vi "gentec-M-Link.Parse Data.vi"(1 "Data Bytes":string, 3 "Measurement":T1 items=["other Mode", "Energymode"]) -> (14 "ADC Counts":u16, 15 "Range":T2 items=["1f", "3f", "10f", "30f", "100f", "300f", "1p", "3p", "10p", "30p", "100p", "300p", "1n", "3n", "10n", "30n", "100n", "300n", "1u", "3u", "10u", "30u", "100u", "300u", "1m", "3m", "10m", "30m", "100m", "300m", "1", "3", "10", "30", "100", "300", "1K", "3K", "10K", "30K", "100K", "300K", "1M", "3M", "10M", "30M", "100M", "300M"], 16 "Pulse Period Counts":u32, 17 "new SSE":bool, 18 "Out":bool)   [LabVIEW 2014, in "gentec-M-Link - Driver.lvlib"]
uses:
  gentec-M-Link - Driver.lvlib
  Type Defs/gentec-M-Link.Range.ctl
  Type Defs/gentec-M-Link.Measurement Mode.ctl
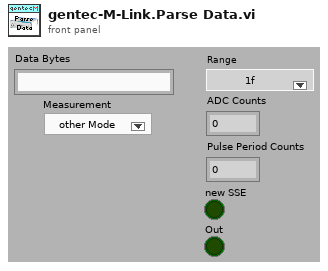
[diagram p1: front panel]
types:
  T1 = typedef "gentec-M-Link - Driver.lvlib/gentec-M-Link.Measurement Mode.ctl" = u16
  T2 = typedef "gentec-M-Link - Driver.lvlib/gentec-M-Link.Range.ctl" = u16
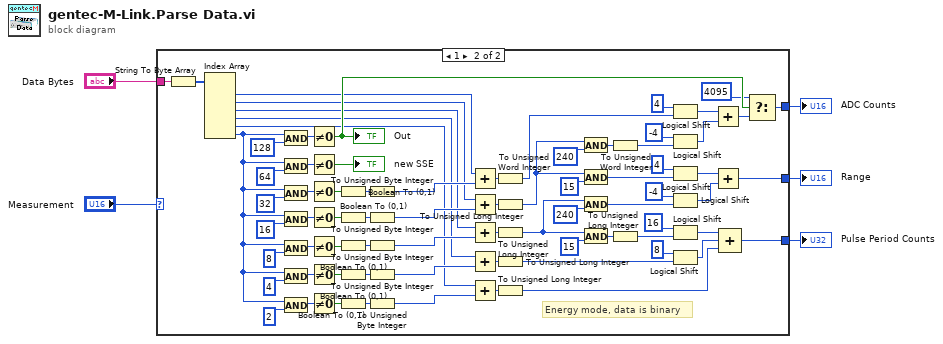
[diagram p0: block diagram]
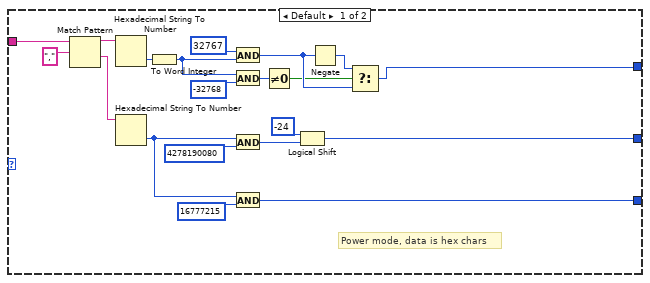
[diagram p2: hidden frame]
diagram:
  n1 = case shown="1" "Measurement" {
    tunnel: [w17 w100] -> w3
    tunnel: [w8 w99] -> w1
    tunnel: [w7 w101] -> w2
    tunnel: "Data Bytes" -> [w6 w98]
    frame Default {
      # "Power mode, data is hex chars"
      n2 = Match Pattern(string=w6, regular expression=",") -> (before substring=w24:string, after substring=w23:string)  [unwired: 3 out]
      n3 = Hexadecimal String To Number(string=w24) -> (number=w9:u32)  [unwired: 3 out]
      n4 = Hexadecimal String To Number(string=w23) -> (number=w21:u32)  [unwired: 3 out]
      n5 = To Word Integer(number=w9) -> (16bit integer=w16:i16)
      n6 = And(x=i16 32767 ("y"), y=w16) -> (x .and. y?=w15:i16)
      n7 = And(x=w16, y=i16 -32768) -> (x .and. y?=w11:i16)
      n8 = And(x=w21, y=u32 4278190080) -> (x .and. y?=w19:u32)
      n9 = And(x=w21, y=u32 16777215) -> (x .and. y?=w8:u32)
      n10 = Not Equal To 0?(x=w11) -> (x != 0?=w13:bool)
      n11 = Logical Shift(y=i8 -24, x=w19) -> (x << y=w7:u32)
      n12 = Negate(x=w15) -> (-x=w14:i16)
      n13 = Select(t=w14, s=w13, f=w15) -> (s? t:f=w17:i16)
    }
    frame 1 {
      # "Energy mode, data is binary"
      n14 = String To Byte Array(string=w98) -> (unsigned byte array=w66:u8[])
      n15 = Index Array(array=w66) -> (element #1=w33:u8, element #2=w30:u8, element #3=w29:u8, element #4=w28:u8, element #5=w26:u8, element #6=w27:u8)  [unwired: 6 in]
      n16 = And(x=w27, y=u8 128) -> (x .and. y?=w90:u8)
      n17 = And(x=w27, y=u8 64) -> (x .and. y?=w73:u8)
      n18 = And(x=w27, y=u8 32) -> (x .and. y?=w88:u8)
      n19 = And(x=w27, y=u8 16) -> (x .and. y?=w86:u8)
      n20 = And(x=w27, y=u8 8) -> (x .and. y?=w82:u8)
      n21 = And(x=w27, y=u8 4) -> (x .and. y?=w80:u8)
      n22 = And(x=w27, y=u8 2) -> (x .and. y?=w76:u8)
      n23 = Not Equal To 0?(x=w90) -> (x != 0?=w97:bool)
      "Out" <- w97
      n24 = Not Equal To 0?(x=w73) -> (x != 0?=→"new SSE":bool)
      n25 = Not Equal To 0?(x=w88) -> (x != 0?=w85:bool)
      n26 = Not Equal To 0?(x=w86) -> (x != 0?=w84:bool)
      n27 = Not Equal To 0?(x=w82) -> (x != 0?=w79:bool)
      n28 = Not Equal To 0?(x=w80) -> (x != 0?=w78:bool)
      n29 = Not Equal To 0?(x=w76) -> (x != 0?=w75:bool)
      n30 = Boolean To (0,1)(Boolean=w85) -> (0, 1=w71:i16)
      n31 = Boolean To (0,1)(Boolean=w84) -> (0, 1=w70:i16)
      n32 = Boolean To (0,1)(Boolean=w79) -> (0, 1=w69:i16)
      n33 = Boolean To (0,1)(Boolean=w78) -> (0, 1=w68:i16)
      n34 = Boolean To (0,1)(Boolean=w75) -> (0, 1=w67:i16)
      n35 = To Unsigned Byte Integer(number=w71) -> (unsigned 8bit integer=w96:u8)
      n36 = To Unsigned Byte Integer(number=w70) -> (unsigned 8bit integer=w95:u8)
      n37 = To Unsigned Byte Integer(number=w69) -> (unsigned 8bit integer=w94:u8)
      n38 = To Unsigned Byte Integer(number=w68) -> (unsigned 8bit integer=w93:u8)
      n39 = To Unsigned Byte Integer(number=w67) -> (unsigned 8bit integer=w92:u8)
      n40 = Add(x=w33, y=w96) -> (x+y=w40:u8)
      n41 = Add(x=w30, y=w95) -> (x+y=w37:u8)
      n42 = Add(x=w29, y=w94) -> (x+y=w35:u8)
      n43 = Add(x=w28, y=w93) -> (x+y=w39:u8)
      n44 = Add(x=w26, y=w92) -> (x+y=w38:u8)
      n45 = To Unsigned Word Integer(number=w40) -> (unsigned 16bit integer=w51:u16)
      n46 = To Unsigned Long Integer(number=w37) -> (unsigned 32bit integer=w36:u32)
      n47 = To Unsigned Long Integer(number=w35) -> (unsigned 32bit integer=w34:u32)
      n48 = To Unsigned Long Integer(number=w39) -> (unsigned 32bit integer=w44:u32)
      n49 = To Unsigned Long Integer(number=w38) -> (unsigned 32bit integer=w41:u32)
      n50 = And(x=w36, y=u8 240) -> (x .and. y?=w50:u32)
      n51 = And(x=w36, y=u8 15) -> (x .and. y?=w57:u32)
      n52 = And(x=w34, y=u8 240) -> (x .and. y?=w56:u32)
      n53 = And(x=w34, y=u8 15) -> (x .and. y?=w48:u32)
      n54 = To Unsigned Word Integer(number=w50) -> (unsigned 16bit integer=w49:u16)
      n55 = To Unsigned Long Integer(number=w48) -> (unsigned 32bit integer=w46:u32)
      n56 = Logical Shift(y=i8 4, x=w51) -> (x << y=w52:u16)
      n57 = Logical Shift(y=i8 -4, x=w49) -> (x << y=w53:u16)
      n58 = Logical Shift(y=i8 4, x=w57) -> (x << y=w63:u32)
      n59 = Logical Shift(y=i8 -4, x=w56) -> (x << y=w62:u32)
      n60 = Logical Shift(y=i8 16, x=w46) -> (x << y=w43:u32)
      n61 = Logical Shift(y=i8 8, x=w44) -> (x << y=w42:u32)
      n62 = Add(x=w52, y=w53) -> (x+y=w32:u16)
      n63 = Add(x=w63, y=w62) -> (x+y=w101:u32)
      n64 = Compound Arithmetic op=ADD(w43, w42, w41) -> (w99:u32)
      n65 = Select(t=u16 4095, s=w97, f=w32) -> (s? t:f=w100:u16)
    }
  }
  "ADC Counts" <- w3
  "Range" <- w2
  "Pulse Period Counts" <- w1
